vi "QueryPNInfo.vi"(0 "PN":string="cn07tpNW748701C2001KX03") -> (21 "Data":string[](array[string]), 24 "Query Result":bool)   [LabVIEW 2011]
panel:
  in  "Excel._Application":refnum<k7>
  in  "Excel._Worksheet":refnum<k7>
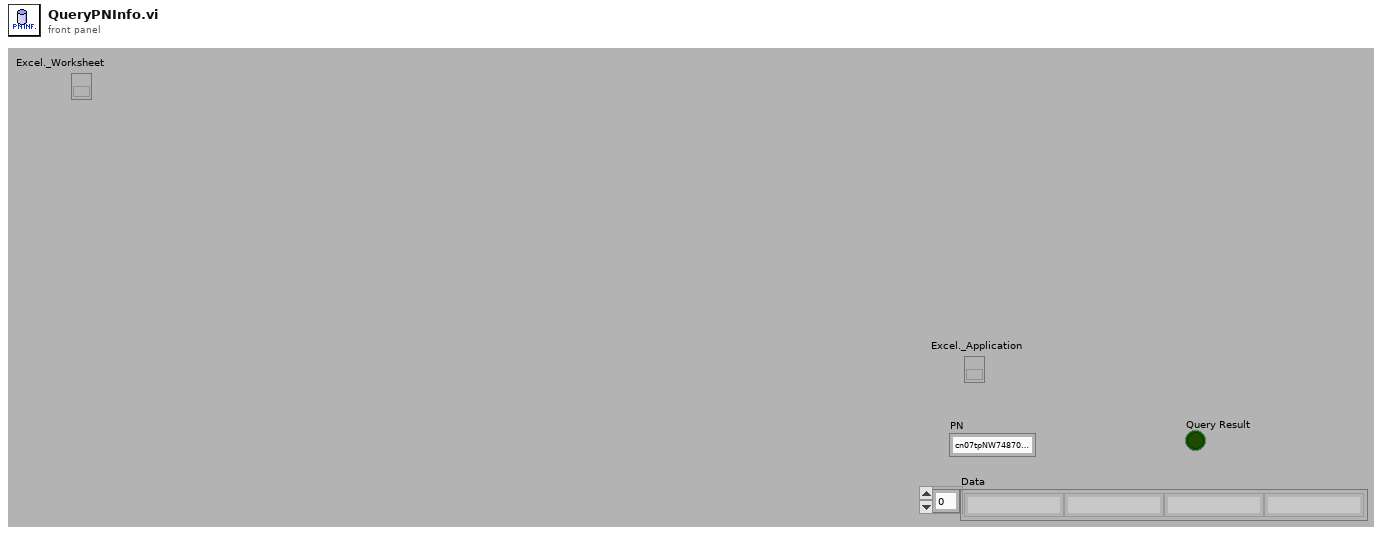
[diagram p1: front panel]
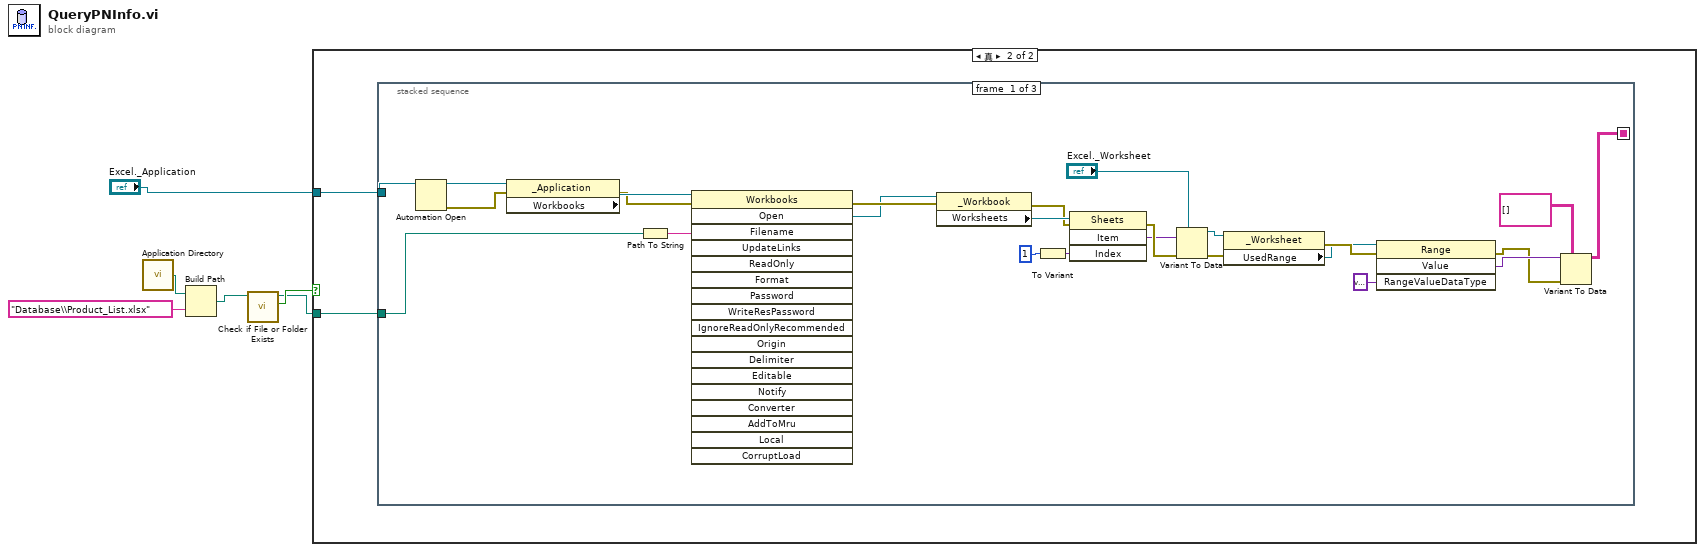
[diagram p0: block diagram]
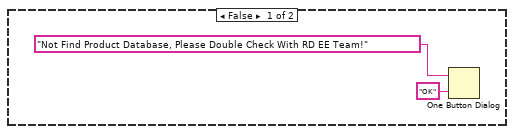
[diagram p2: hidden frame]
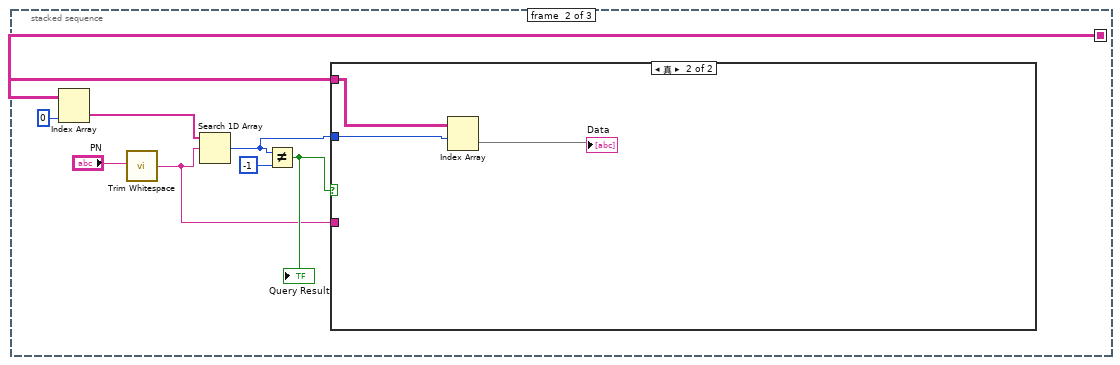
[diagram p3: hidden frame]
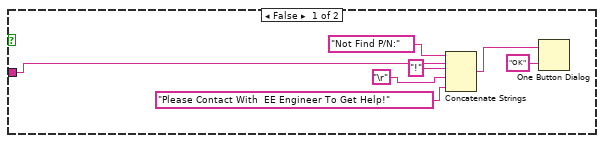
[diagram p4: hidden frame]
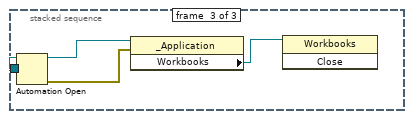
[diagram p5: hidden frame]
diagram:
  n1 = call <vilib>:"Application Directory.vi"() -> ("Application Directory"=w5:path)
  n2 = Build Path(base path=w5, name or relative path="Database\\Product_List.xlsx" ("名称或相对路径")) -> (appended path=w3:path)
  n3 = call <vilib>:"Check if File or Folder Exists.vi"("path"=w3) -> ("file or folder exists?"=w2:bool, "dup path"=w1:path)  [unwired: 8 in, 1 out]
  n4 = case shown="真" w2 {
    tunnel: "Excel._Application" -> [_ w10]
    tunnel: w1 -> [_ w9]
    frame False {
      n5 = One Button Dialog(message="Not Find Product Database, Please Double Check With RD EE Team!" ("消息"), button name ("OK")="OK" ("按钮名称（“确定”）")) -> ()  [unwired: 1 out]
    }
    frame True {
      n6 = stacked-sequence {
        seq-local: [w11 _ _] -> [_ w37 _]
        tunnel: w10 -> [w12 _ w55]
        tunnel: w9 -> [w17 _ _]
        frame #0 {
          n7 = Automation Open(Automation Refnum=w12) -> (Automation Refnum=w13:refnum<k7>, error out=w35:errorcluster)  [unwired: 3 in]
          n8 = property class="_Application"(reference=w13, error in=w35) -> (error out=w33:errorcluster, "Workbooks"=w34:refnum<k7>)  [unwired: 1 out]
          n9 = Path To String(path=w17) -> (string=w16:string)
          n10 = invoke class="Workbooks" method="Open"(reference=w34, error in=w33, "Filename"=w16) -> (error out=w32:errorcluster, "Open"=w14:refnum<k7>)  [unwired: 15 in, 16 out]
          n11 = property class="_Workbook"(reference=w14, error in=w32) -> (error out=w27:errorcluster, "Worksheets"=w31:refnum<k7>)  [unwired: 1 out]
          n12 = To Variant(anything=1) -> (Variant=w29:variant)
          n13 = invoke class="Sheets" method="Item"(reference=w31, error in=w27, "Index"=w29) -> (error out=w28:errorcluster, "Item"=w26:variant)  [unwired: 1 in, 2 out]
          n14 = Variant To Data(error in=w28, type="Excel._Worksheet", Variant=w26) -> (data=w24:refnum<k7>, error out=w23:errorcluster)
          n15 = property class="_Worksheet"(reference=w24, error in=w23) -> (error out=w20:errorcluster, "UsedRange"=w15:refnum<k7>)  [unwired: 1 out]
          n16 = invoke class="Range" method="Value"(reference=w15, error in=w20, "RangeValueDataType"=variant) -> (error out=w18:errorcluster, "Value"=w22:variant)  [unwired: 1 in, 2 out]
          n17 = Variant To Data(error in=w18, type=string[][] [] ("添加的数组"), Variant=w22) -> (data=w11:string[][])  [unwired: 1 out]
        }
        frame #1 {
          n18 = Index Array(array=w37, index (col)=0 ("禁用的索引 (列)")) -> (element=w42:string[])  [unwired: 1 in]
          n19 = call <vilib>:"Trim Whitespace.vi"("string"="PN") -> ("trimmed string"=w38:string)  [unwired: 1 in]
          n20 = Search 1D Array(1D array=w42, element=w38) -> (index of element=w36:i32)  [unwired: 1 in]
          n21 = Not Equal?(x=w36, y=-1) -> (x != y?=w39:bool)
          "Query Result" <- w39
          n22 = case shown="真" w39 {
            tunnel: w38 -> [w46 _]
            tunnel: w37 -> [_ w53]
            tunnel: w36 -> [_ w52]
            frame False {
              n23 = Concatenate Strings("Not Find P/N:" ("消息"), w46, "!" ("字符串"), "\r", "Please Contact With  EE Engineer To Get Help!" ("字符串")) -> (w48:string)
              n24 = One Button Dialog(message=w48, button name ("OK")="OK" ("按钮名称（“确定”）")) -> ()  [unwired: 1 out]
            }
            frame True {
              n25 = Index Array(array=w53, index (row)=w52) -> (element=→"Data":string[])  [unwired: 1 in]
            }
          }
        }
        frame #2 {
          n26 = Automation Open(Automation Refnum=w55) -> (Automation Refnum=w56:refnum<k7>, error out=w57:errorcluster)  [unwired: 3 in]
          n27 = property class="_Application"(reference=w56, error in=w57) -> ("Workbooks"=w54:refnum<k7>)  [unwired: 2 out]
          n28 = invoke class="Workbooks" method="Close"(reference=w54) -> ()  [unwired: 2 in, 3 out]
        }
      }
    }
  }
